vi "add time stamp.vi"(2 "delta x":dbl=0.05 format="%.5f", 3 "signal 1":dbl[](array[numeric])) -> (1 "Data w time":ext[][](array[numeric]) format="%#.2f")   [LabVIEW 2010]
panel:
  out "extended precision float":ext format="%#.2f"
  out "current time":timestamp
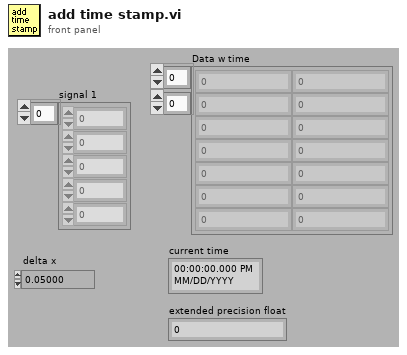
[diagram p1: front panel]
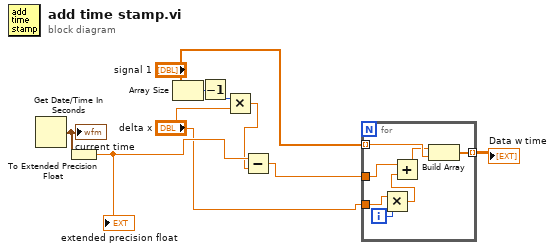
[diagram p0: block diagram]
diagram:
  n1 = Get Date/Time In Seconds() -> (seconds since 1Jan1904=w9:timestamp)
  "current time" <- w9
  n2 = To Extended Precision Float(1:w9) -> (0:w6:ext)
  "extended precision float" <- w6
  n3 = Array Size(array="signal 1") -> (size(s)=w7:i32)
  n4 = Decrement(x=w7) -> (x-1=w4:i32)
  n5 = Multiply(x=w4, y="delta x") -> (x*y=w2:dbl)
  n6 = Subtract(x=w6, y=w2) -> (x-y=w3:ext)
  n7 = for {
    tunnel: "signal 1" -> [w11] mode=indexing
    tunnel: w3 -> [w13]
    tunnel: [w14] -> w5 mode=indexing
    tunnel: "delta x" -> [w12]
    i -> [w15]
    n8 = Multiply(x=w12, y=w15) -> (x*y=w16:dbl)
    n9 = Add(x=w13, y=w16) -> (x+y=w10:ext)
    n10 = Build Array(w10, w11) -> (w14:ext[])
  }
  "Data w time" <- w5
